vi "OFBS_writeClassifierParam.vi"(6 "Quality Measure in":T1, 8 "error in (no error)":errorcluster, 9 "Metaparameter in":dbl, 10 "Classifier Type in":T2, 11 "OptFreqBandsSearch in":refnum<class "OptFreqBandsSearch.lvclass">) -> (0 "error out":errorcluster, 3 "OptFreqBandsSearch out":refnum<class "OptFreqBandsSearch.lvclass">)   [LabVIEW 2016, in "Optimal Frequency Bands Search.lvlib" / "OptFreqBandsSearch.lvclass"]
uses:
  OptFreqBandsSearch.lvclass
  4. Accuracy Assessment for EEG Classification/_vlib/CU_ClassifierTypes.ctl
  4. Accuracy Assessment for EEG Classification/_vlib/CU_ClassifierQualityMeasure.ctl
  OptFreqBandsSearch.lvclass/OptFreqBandsSearch.ctl
  4. Accuracy Assessment for EEG Classification/Classifier.lvlib
panel:
  # "This VI is a part of BCI Design library, http://www.ru-bci.org \nCopyright © 2020, Sotnikov Peter, All rights reserved. License: CC BY-NC 4.0"
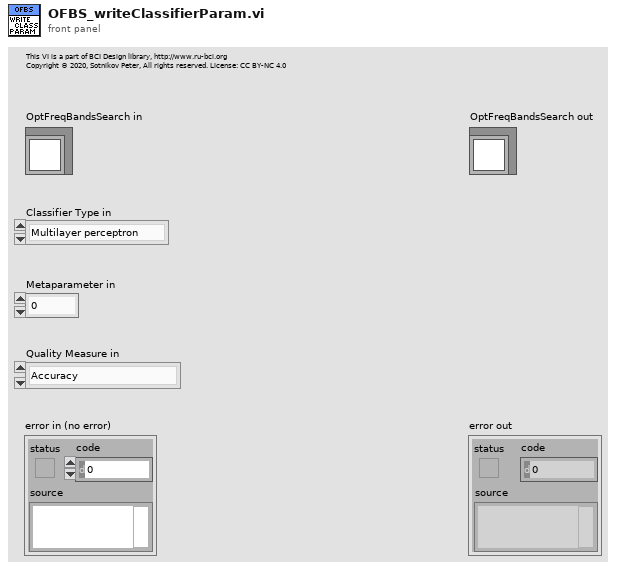
[diagram p1: front panel]
types:
  T1 = typedef "Classifier.lvlib/CU_ClassifierQualityMeasure.ctl" = enum16{"Accuracy", "Cohen's kappa"}
  T2 = typedef "Classifier.lvlib/CU_ClassifierTypes.ctl" = enum16{"Multilayer perceptron", "k NN Classifier", "SVM Committee", "Mahalanobis distance", "SVM Classifier"}
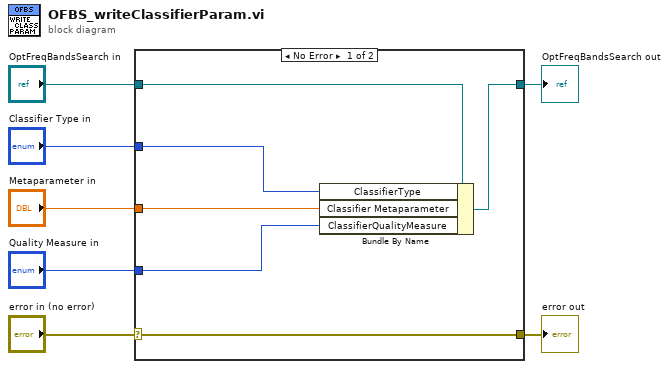
[diagram p0: block diagram]
diagram:
  n1 = case shown="No Error" "error in (no error)" {
    selector: "error in (no error)" -> [w13 w14]
    tunnel: [w13 w14] -> w6
    tunnel: [w11 w15] -> w4
    tunnel: "OptFreqBandsSearch in" -> [w12 w15]
    tunnel: "Classifier Type in" -> [w10 _]
    tunnel: "Metaparameter in" -> [w8 _]
    tunnel: "Quality Measure in" -> [w9 _]
    frame No Error {
      n2 = Bundle By Name(cluster=w12, "ClassifierType"=w10, "Classifier Metaparameter"=w8, "ClassifierQualityMeasure"=w9) -> (w11:refnum<class "OptFreqBandsSearch.lvclass">)
    }
    frame Error {
    }
  }
  "error out" <- w6
  "OptFreqBandsSearch out" <- w4
